vi "CallReadTDCHit.vi"(8 "error in (no error)":errorcluster, 9 "data value reference":T2, 11 ".NET Refnum in":T3) -> (0 "error out":errorcluster, 1 "data value reference out":T2, 2 "# of hits read":i32, 3 ".NET Refnum out":T3, 4 "Array":T1[](array[typedef]))   [LabVIEW 2016, in "HPTDC Driver Library.lvlib"]
uses:
  HPTDC Driver Library.lvlib
  Typedefs/TDCManager.ctl
  C:/Users/CRT Controller/CRTC Labview Application/Source/HPTDC Driver Library Folder/Library files/hptdc_net4_3.7.0_x64.dll
  hptdc_net4_3.7.0_x64.dll
  Typedefs/TDCHitArrayPointer.ctl
  Typedefs/TDCHit.ctl
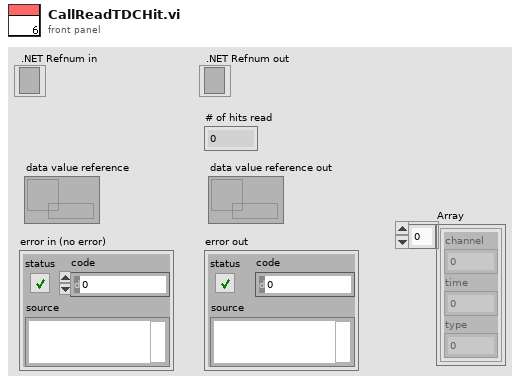
[diagram p1: front panel]
types:
  T1 = typedef "HPTDC Driver Library.lvlib/TDCHit.ctl" = cluster{"channel":u8, "time":u64, "type":u8}
  T2 = typedef "TDCHitArrayPointer.ctl" = refnum<data-value>
  T3 = typedef "HPTDC Driver Library.lvlib/TDCManager.ctl" = refnum<k24>
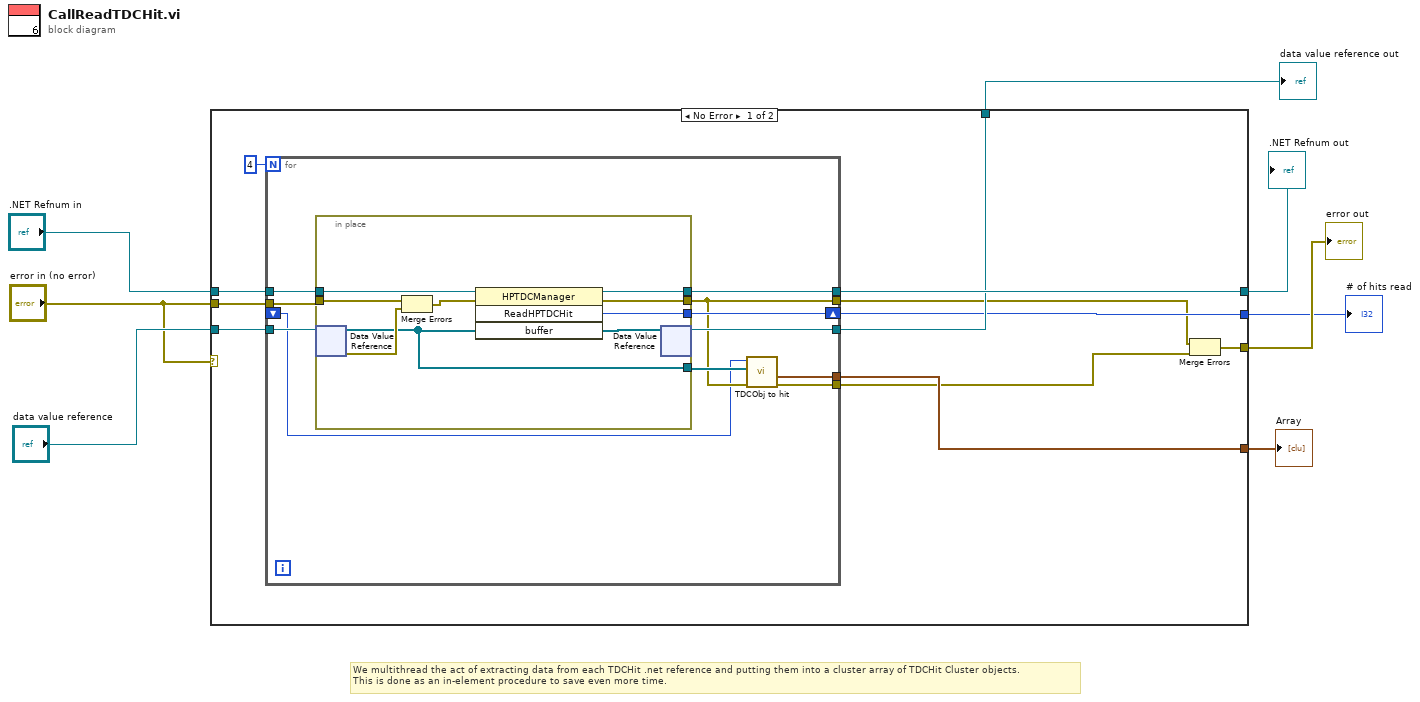
[diagram p0: block diagram]
diagram:
  # "We multithread the act of extracting data from each TDCHit .net reference and putting them into a cluster array of TDCHit Cluster objects.\nThis is done as an in-element procedure to save even more time."
  n1 = case shown="No Error" "error in (no error)" {
    tunnel: [w19 w42] -> w8
    tunnel: ".NET Refnum in" -> [w18 w42]
    tunnel: "error in (no error)" -> [w17 w40]
    tunnel: [w16 w40] -> w6
    tunnel: [w15 w41] -> w5
    tunnel: "data value reference" -> [w14 w41]
    tunnel: [w13 _] -> w3
    tunnel: [w12 _] -> w2
    frame No Error {
      n2 = for {
        N: 4 -> [_]
        tunnel: [w30] -> w19
        tunnel: w18 -> [w29]
        tunnel: w17 -> [w28]
        tunnel: [w27] -> w15
        tunnel: w14 -> [w26]
        tunnel: [w23] -> w12
        tunnel: [w22] -> w11
        tunnel: [w21] -> w10
        shift-right: [w24] -> w13
        shift-left: _ -> [w20]
        n3 = in-place {
          in-place-border: [w32] -> w24
          in-place-border: [w39] -> w30
          in-place-border: [w34] -> w21
          in-place-border: w29 -> [w38]
          in-place-border: w28 -> [w35]
          in-place-border: [w33] -> w25
          n4 = in-place-dvr #1(w26) -> (w33:refnum<k24>[], w36:errorcluster)
          n5 = Merge Errors(w35, w36) -> (w37:errorcluster)
          n6 = invoke class="HPTDCManager" method="ReadHPTDCHit"(reference=w38, error in=w37, "buffer"=w33) -> (reference out=w39:T3, error out=w34:errorcluster, "ReadHPTDCHit"=w32:i32, "buffer"=w31:refnum<k24>[])  [unwired: 1 in]
          n7 = in-place-dvr #1(w31) -> (w27:T2)  [unwired: 1 out]
        }
        n8 = call "TDCObj to hit.vi"("error in"=w21, "TDCHits Buffer"=w25, "#of hits"=w20) -> ("error out"=w22:errorcluster, "Array"=w23:T1[])  [unwired: 7 in]
      }
      n9 = Merge Errors(w10, w11) -> (w16:errorcluster)
    }
    frame Error {
    }
  }
  "# of hits read" <- w3
  ".NET Refnum out" <- w8
  "error out" <- w6
  "data value reference out" <- w5
  "Array" <- w2
